vi "Drive PID.vi"(11 "Process Variable":dbl format="%.2f") -> (3 "Output":dbl format="%.2f")   [LabVIEW 2014]
uses:
  <vilib>/Rock Robotics/WPI/DriverStation/WPI_DriverStationRobotMode2.ctl
  Robot Global Data.vi
  <vilib>/addons/control/pid/pid.llb/PID (DBL).vi
  <vilib>/addons/control/pid/NI_PID_pid.lvlib
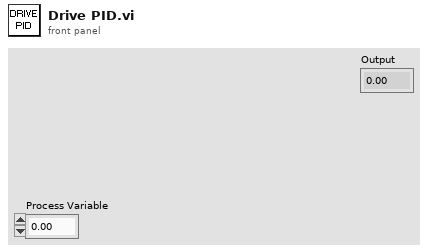
[diagram p1: front panel]
types:
  T1 = typedef "WPI_DriverStationRobotMode2.ctl" = enum16{"Autonomous Disabled", "Autonomous Enabled", "Teleop Disabled", "Teleop Enabled", "Disconnected", "Finish", "Test Disabled", "Test Enabled", "Emergency Stopped"}
  T2 = cluster{"proportional gain (Kc)":dbl, "integral time (Ti, min)":dbl, "derivative time (Td, min)":dbl}
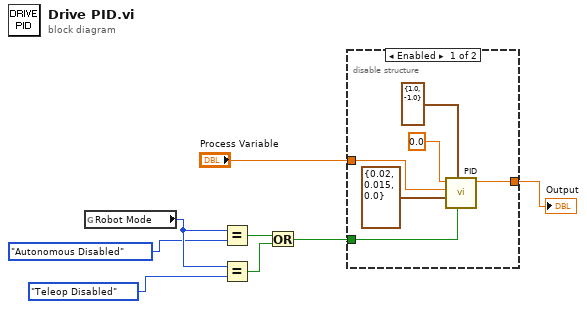
[diagram p0: block diagram]
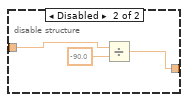
[diagram p2: hidden frame]
diagram:
  n1 = global read "Robot Global Data.vi" "Robot Mode"() -> (w3:T1)
  n2 = Equal?(x=w3, y=WPI_DriverStationRobotMode2."Autonomous Disabled" ("Robot Mode")) -> (x = y?=w6:bool)
  n3 = Equal?(x=w3, y=WPI_DriverStationRobotMode2."Teleop Disabled" ("Robot Mode")) -> (x = y?=w5:bool)
  n4 = Or(x=w6, y=w5) -> (x .or. y?=w4:bool)
  n5 = disable-structure shown="Enabled" {
    disable-tunnel: "Process Variable" -> [w11 w16]
    disable-tunnel: [w10 w15] -> w7
    disable-tunnel: w4 -> [w9 _]
    frame Enabled {
      n6 = call-poly <vilib>:"PID.vi"("reinitialize? (F)"=w9, "output range"=cluster{"output high":dbl, "output low":dbl} {"output high"=1.0, "output low"=-1.0}, "PID gains"=T2 {"proportional gain (Kc)"=0.02, "integral time (Ti, min)"=0.015, "derivative time (Td, min)"=0.0}, "process variable"=w11, "setpoint"=0.0) -> ("output"=w10:dbl)  [unwired: 5 in, 1 out]
    }
    frame Disabled {
      n7 = Divide(x=w16, y=-90.0) -> (x/y=w15:dbl)
    }
  }
  "Output" <- w7
